vi "Read Spec Page Path.vi"(8 "error in":errorcluster, 11 "decideprojectfeatures in":refnum<class "SequencerActionScript.lvclass">) -> (0 "error out":errorcluster, 2 "path to spec page vi":path, 3 "decideprojectfeatures out":refnum<class "SequencerActionScript.lvclass">)   [LabVIEW 2014, in "SequencerActionScript.lvclass"]
doc: "NI Tag Bus Module Framework 1.0.2.36\nNI Systems Engineering"
uses:
  SequencerActionScript.lvclass
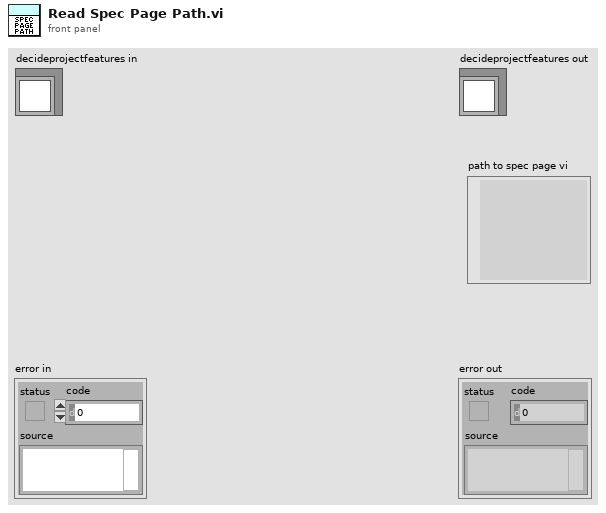
[diagram p1: front panel]
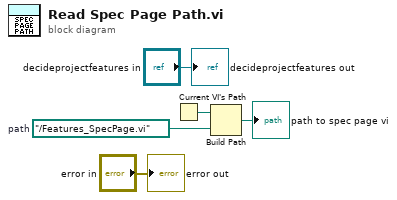
[diagram p0: block diagram]
diagram:
  w2 = path "../Features_SpecPage.vi"  # path
  n1 = Current VI's Path() -> (path=w3:path)
  n2 = Build Path(base path=w3, name or relative path=w2) -> (appended path=→"path to spec page vi":path)
  "error out" <- "error in"
  "decideprojectfeatures out" <- "decideprojectfeatures in"
